vi "Stop Core.vi"(10 "final error code":i32 caption="最终错误代码", 11 "P3AT in":refnum<class "RemoteP3AT.lvclass"> caption="操作者输入") -> (3 "P3AT out":refnum<class "RemoteP3AT.lvclass"> caption="操作者输出")   [LabVIEW 2014, in "RemoteP3AT.lvlib" / "RemoteP3AT.lvclass"]
doc: "(<B>文件名</B>：Actor Framework.lvlib:Actor.lvclass:Stop Core.vi)\n\n定义停止前操作者的动作。使用<B>最终错误代码</B>输入判断操作者是否在出错时关闭。\n\n默认情况下，该方法不执行任何动作。子孙类重写该方法，定义出错时的操作，例如，关闭操作者核心方法初始的进程。"
uses:
  RemoteP3AT.lvclass
  RemoteP3AT.lvclass/RemoteP3AT.ctl
  Wrapper_lib/zsActor/ActorWrapper.lvclass
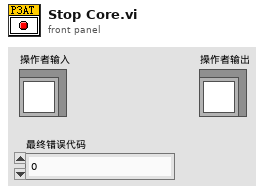
[diagram p1: front panel]
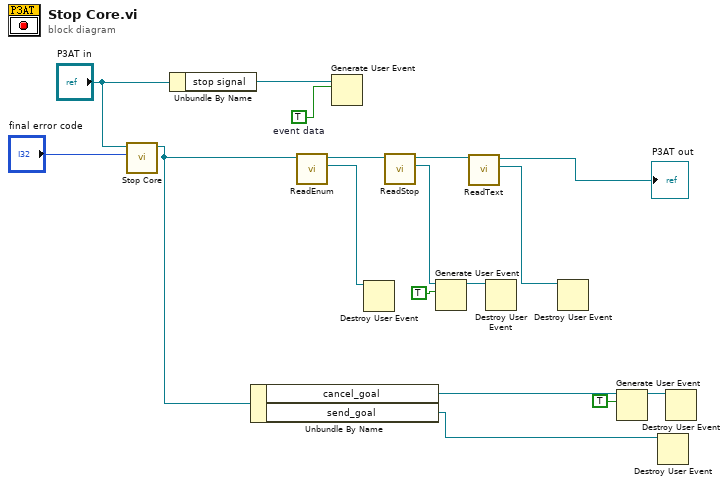
[diagram p0: block diagram]
diagram:
  w15 = TRUE  # event data
  n1 = call-parent "Stop Core.vi"("final error code"="final error code", "Actor in"="P3AT in") -> ("Actor out"=w3:refnum<class "RemoteP3AT.lvclass">)  [unwired: 9 in]
  n2 = Unbundle By Name("P3AT in") -> ("stop signal"=w14:refnum<user-event>)
  n3 = Unbundle By Name(w3) -> ("cancel_goal"=w13:refnum<user-event>, "send_goal"=w1:refnum<user-event>)
  n4 = call-dynamic "ReadEnum.vi"("zsActor输入"=w3) -> ("Enum"=w6:refnum<user-event>, "zsActor输出"=w10:refnum<class "RemoteP3AT.lvclass">)  [unwired: 8 in, 1 out]
  n5 = Generate User Event(user event=w14, event data cluster=w15) -> ()  [unwired: 2 in, 2 out]
  n6 = Destroy User Event(user event=w6) -> ()  [unwired: 1 in, 1 out]
  n7 = call-dynamic "ReadStop.vi"("zsActor输入"=w10) -> ("Stop"=w5:refnum<user-event>, "zsActor输出"=w9:refnum<class "RemoteP3AT.lvclass">)  [unwired: 8 in, 1 out]
  n8 = Generate User Event(user event=w5, event data cluster=TRUE ("event data")) -> (user event out=w7:refnum<user-event>)  [unwired: 2 in, 1 out]
  n9 = call-dynamic "ReadText.vi"("zsActor输入"=w9) -> ("Text"=w4:refnum<user-event>, "zsActor输出"=→"P3AT out":refnum<class "RemoteP3AT.lvclass">)  [unwired: 8 in, 1 out]
  n10 = Destroy User Event(user event=w7) -> ()  [unwired: 1 in, 1 out]
  n11 = Destroy User Event(user event=w4) -> ()  [unwired: 1 in, 1 out]
  n12 = Generate User Event(user event=w13, event data cluster=TRUE ("event data")) -> (user event out=w11:refnum<user-event>)  [unwired: 2 in, 1 out]
  n13 = Destroy User Event(user event=w1) -> ()  [unwired: 1 in, 1 out]
  n14 = Destroy User Event(user event=w11) -> ()  [unwired: 1 in, 1 out]
